vi "Timed Setpoint.vi"(8 "Cycle count":dbl, 11 "Setpoint In":dbl) -> (3 "Setpoint Out":dbl)   [LabVIEW 2025]
uses:
  ef10dad4-8f2e-4dc8-93cb-ed4b71121f5a.vi
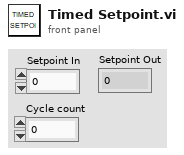
[diagram p1: front panel]
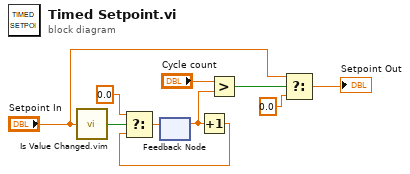
[diagram p0: block diagram]
diagram:
  n1 = call "Is Value Changed.vim"("value"="Setpoint In") -> ("changed or first call?"=w10:bool)
  n2 = feedback #1() -> (w6:dbl)  [unwired: 1 in]
  n3 = Increment(x=w6) -> (x+1=w7:dbl)
  n4 = Select(t=0.0, s=w10, f=w7) -> (s? t:f=w8:dbl)
  n5 = feedback-in #1(w8) -> ()
  n6 = Greater?(x="Cycle count", y=w6) -> (0:w4:bool)
  n7 = Select(t="Setpoint In", s=w4, f=0.0) -> (s? t:f=→"Setpoint Out":dbl)
